vi "BoxDashRead.vi"   [LabVIEW 2023]
uses:
  <vilib>/Rock Robotics/Network Tables/NT Read Number.vi
  BoxGlobals.vi
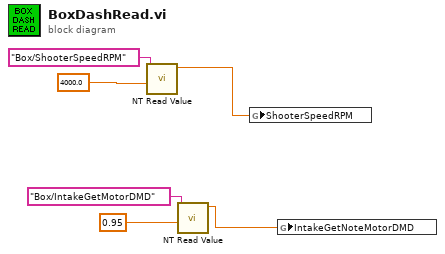
[diagram p0: block diagram]
diagram:
  n1 = call-poly <vilib>:"NT Read Value.vi"("default value"=4000.0, "name"="Box/ShooterSpeedRPM") -> ("value"=w2:dbl)  [unwired: 7 in, 2 out]
  n2 = call-poly <vilib>:"NT Read Value.vi"("default value"=0.95, "name"="Box/IntakeGetMotorDMD") -> ("value"=w1:dbl)  [unwired: 7 in, 2 out]
  n3 = global write "BoxGlobals.vi" "ShooterSpeedRPM"(w2) -> ()
  n4 = global write "BoxGlobals.vi" "IntakeGetNoteMotorDMD"(w1) -> ()
